vi "Simple pulse sweep.vi"() -> ()   [LabVIEW 2019]
uses:
  <instrlib>/LV_PulseRiderPG1000/Public/Configure/Trigger/Trigger Source.ctl
  <instrlib>/LV_PulseRiderPG1000/Public/Configure/Trigger/Trigger Mode.ctl
  <instrlib>/LV_PulseRiderPG1000/Public/Configure/Pulse/Pulse Mode.ctl
  <vilib>/Analysis/1siggen.llb/Ramp Pattern by Delta.vi
  <instrlib>/LV_PulseRiderPG1000/Pulse Rider PG-1000.lvlib
  <vilib>/Analysis/NI_AALBase.lvlib
panel:
  in  "channel":i32=1 min=1 max=4
  in  "pulse width (s)":dbl=1e-09 min=0.005 max=5.0
  in  "step (V)":dbl=0.1
  in  "end (V)":dbl=2.5 min=-5.0 max=5.0 format="%#_6p"
  in  "start (V)":dbl=-2.5 min=-5.0 max=5.0 format="%#_6p"
  out "error out":errorcluster
  in  "VISA resource name":refnum<visa-resource-name>="PG-AT"
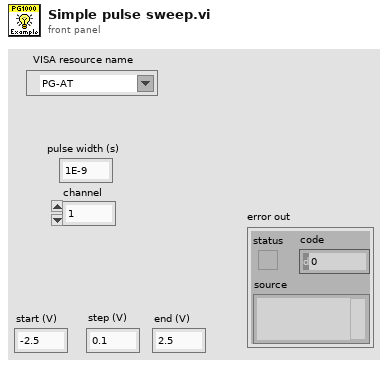
[diagram p1: front panel]
types:
  T1 = typedef "Pulse Rider PG-1000.lvlib/Pulse Mode.ctl" = u16
  T2 = typedef "Pulse Rider PG-1000.lvlib/Trigger Mode.ctl" = u16
  T3 = typedef "Pulse Rider PG-1000.lvlib/Trigger Source.ctl" = enum16{"Manual", "External", "Timer"}
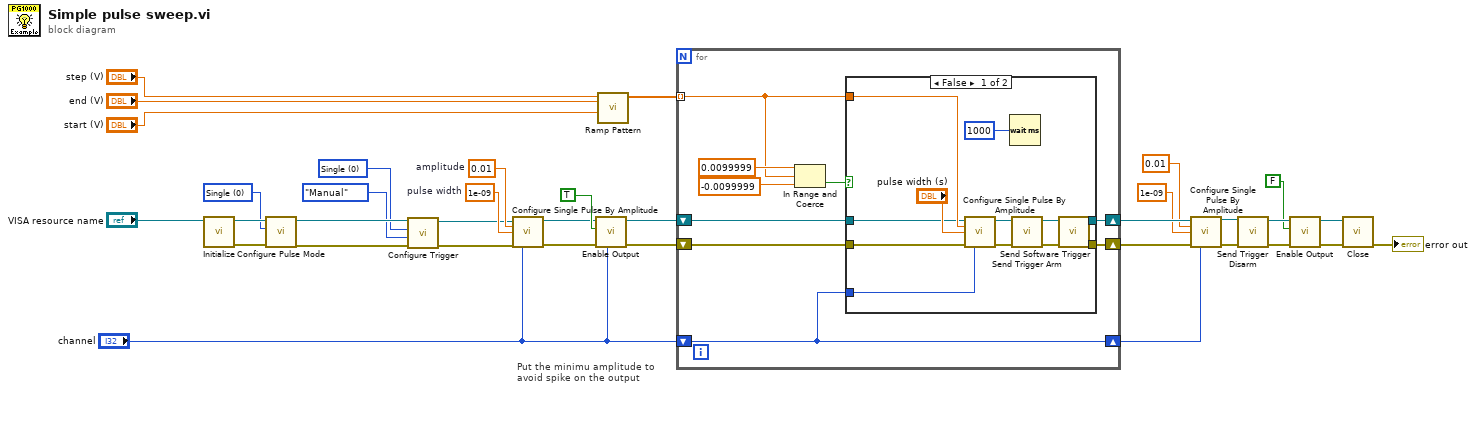
[diagram p0: block diagram]
diagram:
  w5 = T1 0 items=["Single", "Double", "Triple", "Quadruple", "External Width"] ("Pulse Mode (0: single)")
  w6 = T2 0 items=["Single", "Continuous", "Gated", "Burst"] ("mode")
  w31 = 1e-09  # pulse width
  w32 = 0.01  # amplitude
  # "Put the minimu amplitude to avoid spike on the output"
  n1 = call <instrlib>:"Initialize.vi"("VISA resource name"="VISA resource name") -> ("error out"=w29:errorcluster, "VISA resource name out"=w30:refnum<visa-resource-name>)  [unwired: 9 in]
  n2 = call <instrlib>:"Configure Pulse Mode.vi"("error in (no error)"=w29, "Pulse Mode (0: single)"=w5, "VISA resource name"=w30) -> ("error out"=w9:errorcluster, "VISA resource name out"=w11:refnum<visa-resource-name>)  [unwired: 7 in]
  n3 = call <instrlib>:"Configure Trigger.vi"("error in (no error)"=w9, "trigger source"=Trigger_Source."Manual" ("source"), "trigger mode"=w6, "VISA resource name"=w11) -> ("error out"=w8:errorcluster, "VISA resource name out"=w10:refnum<visa-resource-name>)  [unwired: 6 in]
  n4 = call <instrlib>:"Configure Single Pulse By Amplitude.vi"("VISA resource name"=w10, "amplitude (0.01 V)"=w32, "pulse width (s)"=w31, "error in (no error)"=w8, "channel"="channel") -> ("VISA resource name out"=w28:refnum<visa-resource-name>, "error out"=w27:errorcluster)  [unwired: 9 in]
  n5 = call <instrlib>:"Enable Output.vi"("channel"="channel", "error in (no error)"=w27, "Enable Output (T: Enable)"=TRUE, "VISA resource name"=w28) -> ("error out"=w22:errorcluster, "VISA resource name out"=w23:refnum<visa-resource-name>)  [unwired: 6 in]
  n6 = call-poly <vilib>:"Ramp Pattern.vi"("start"="start (V)", "end"="end (V)", "delta"="step (V)") -> ("Ramp Pattern"=w24:dbl[])  [unwired: 6 in, 2 out]
  n7 = for {
    tunnel: w24 -> [w36] mode=indexing
    shift-right: [w41] -> w18
    shift-left: w22 -> [w43]
    shift-right: [w42] -> w19
    shift-left: w23 -> [w44]
    shift-right: [w40] -> w1
    shift-left: "channel" -> [w40]
    n8 = In Range and Coerce(upper limit=0.0099999, x=w36, lower limit=-0.0099999 ("upper limit")) -> (In Range?=w37:bool)  [unwired: 1 out]
    n9 = case shown="False" w37 {
      tunnel: w36 -> [w54 _]
      tunnel: w44 -> [w52 w57]
      tunnel: w43 -> [w51 w58]
      tunnel: [w48 w57] -> w42
      tunnel: [w47 w58] -> w41
      tunnel: w40 -> [w46 _]
      frame False {
        n10 = call <instrlib>:"Configure Single Pulse By Amplitude.vi"("VISA resource name"=w52, "amplitude (0.01 V)"=w54, "pulse width (s)"="pulse width (s)", "error in (no error)"=w51, "channel"=w46) -> ("VISA resource name out"=w56:refnum<visa-resource-name>, "error out"=w55:errorcluster)  [unwired: 9 in]
        n11 = Wait (ms)(milliseconds to wait=u32 1000) -> ()  [unwired: 1 out]
        n12 = call <instrlib>:"Send Trigger Arm.vi"("error in (no error)"=w55, "VISA resource name"=w56) -> ("error out"=w49:errorcluster, "VISA resource name out"=w50:refnum<visa-resource-name>)  [unwired: 8 in]
        n13 = call <instrlib>:"Send Software Trigger.vi"("error in (no error)"=w49, "VISA resource name"=w50) -> ("error out"=w47:errorcluster, "VISA resource name out"=w48:refnum<visa-resource-name>)  [unwired: 8 in]
      }
      frame True {
      }
    }
  }
  n14 = call <instrlib>:"Configure Single Pulse By Amplitude.vi"("VISA resource name"=w19, "amplitude (0.01 V)"=0.01 ("amplitude (0.005 V)"), "pulse width (s)"=1e-09, "error in (no error)"=w18, "channel"=w1) -> ("VISA resource name out"=w17:refnum<visa-resource-name>, "error out"=w16:errorcluster)  [unwired: 9 in]
  n15 = call <instrlib>:"Send Trigger Disarm.vi"("error in (no error)"=w16, "VISA resource name"=w17) -> ("error out"=w14:errorcluster, "VISA resource name out"=w15:refnum<visa-resource-name>)  [unwired: 8 in]
  n16 = call <instrlib>:"Enable Output.vi"("error in (no error)"=w14, "Enable Output (T: Enable)"=FALSE, "VISA resource name"=w15) -> ("error out"=w3:errorcluster, "VISA resource name out"=w4:refnum<visa-resource-name>)  [unwired: 7 in]
  n17 = call <instrlib>:"Close.vi"("error in (no error)"=w3, "VISA resource name"=w4) -> ("error out"=→"error out":errorcluster)  [unwired: 9 in]
